vi "view ROI already set.vi"(8 "error in (no error)":errorcluster, 11 "ItemTag":string) -> (0 "error out":errorcluster, 3 "intensity plot":u64[][](array[numeric]), 4 "Energy 2d gate out":T1, 6 "which spectrum":string)   [LabVIEW 2016]
doc: "Takes set gates and displays them in the select gating vi"
uses:
  controls/energy 2d selection.ctl
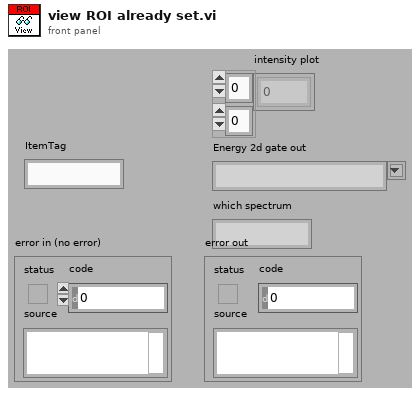
[diagram p1: front panel]
types:
  T1 = typedef "energy 2d selection.ctl" = string
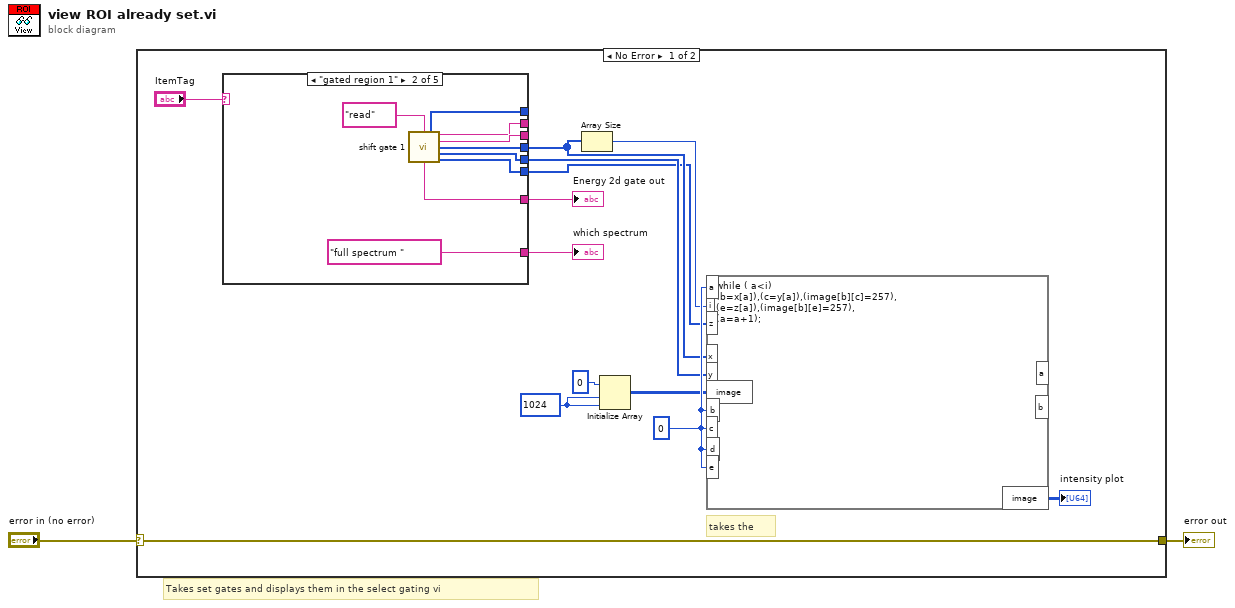
[diagram p0: block diagram]
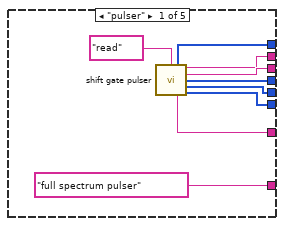
[diagram p2: hidden frame]
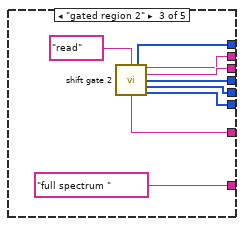
[diagram p3: hidden frame]
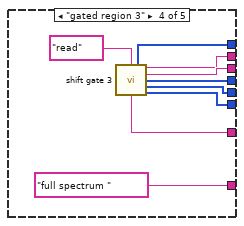
[diagram p4: hidden frame]
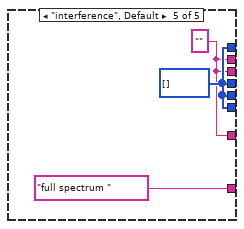
[diagram p5: hidden frame]
diagram:
  # "Takes set gates and displays them in the select gating vi"
  n1 = case shown="No Error" "error in (no error)" {
    selector: "error in (no error)" -> [w10 w55]
    tunnel: [w10 w55] -> w1
    frame No Error {
      w9 = 0 ("input variable")
      w13 = u64 1024 ("dimension size")
      # "takes the"
      n2 = case shown="\"gated region 1\"" "ItemTag" {
        tunnel: [w24 w33 w42 w51 w53] -> _
        tunnel: [w23 w32 w35 w44 w53] -> w14
        tunnel: [w22 w31 w41 w50 w53] -> _
        tunnel: [w21 w30 w40 w49 w54] -> w5
        tunnel: [w20 w29 w39 w48 w54] -> w6
        tunnel: [w19 w28 w38 w47 w54] -> w7
        tunnel: [w17 w26 w36 w45 w54] -> _
        tunnel: ["full spectrum pulser" ("which spectrum") "full spectrum " ("which spectrum") "full spectrum " ("which spectrum") "full spectrum " ("which spectrum") "full spectrum " ("which spectrum")] -> w15
        frame "pulser" {
          n3 = call "shift gate pulser.vi"("shift control"="read") -> ("2d array width output"=w17:i32[], "X name output"=w22:string, "Y name  output"=w24:string, "X range output"=w19:i32[], "Y range Max output"=w20:i32[], "Energy 2d gate out"=w23:T1, "Y range Min output"=w21:i32[])  [unwired: 8 in]
        }
        frame "gated region 1" {
          n4 = call "shift gate 1.vi"("shift control"="read") -> ("2d  array width output"=w26:i32[], "X name output"=w31:string, "Y name  output"=w33:string, "X range output"=w28:i32[], "Y range Max output"=w29:i32[], "Energy 2d gate out"=w32:T1, "Y range Min output"=w30:i32[])  [unwired: 8 in]
        }
        frame "gated region 2" {
          n5 = call "shift gate 2.vi"("shift control"="read") -> ("2d position array output"=w36:i32[], "X name output"=w41:string, "Y name  output"=w42:string, "X range output"=w38:i32[], "Y range Max output"=w39:i32[], "Energy 2d gate out"=w35:T1, "Y range Min output"=w40:i32[])  [unwired: 8 in]
        }
        frame "gated region 3" {
          n6 = call "shift gate 3.vi"("shift control"="read") -> ("2d location array output"=w45:i32[], "X name output"=w50:string, "Y name  output"=w51:string, "X range output"=w47:i32[], "Y range Max output"=w48:i32[], "Energy 2d gate out"=w44:T1, "Y range Min output"=w49:i32[])  [unwired: 8 in]
        }
        frame "interference", Default {
          w54 = i32[] [] ("X range output")
          w53 = "" ("X name output")
        }
      }
      "which spectrum" <- w15
      "Energy 2d gate out" <- w14
      n7 = Array Size(array=w7) -> (size(s)=w8:i32)
      n8 = Initialize Array(u64 0 ("element"), w13, w13) -> (w4:u64[][])
      n9 = formula code="while ( a<i)\n(b=x[a]),(c=y[a]),(image[b][c]=257),\n(e=z[a]),(image[b][e]=257),\n(a=a+1);"("x"=w7, "y"=w6, "image"=w4, "i"=w8, "a"=w9, "b"=w9, "c"=w9, "d"=w9, "e"=w9, "z"=w5) -> ("image"=→"intensity plot":u64[][])  [unwired: 2 out]
    }
    frame Error {
    }
  }
  "error out" <- w1
